vi "kf_update_p_k.vi"(11 "KF in":T2 {"K" format="%#_3g"; "y lim" format="%#_3g"; "x lim" format="%#_3g"; "P" format="%#_3g"; "H" format="%#_3g"; "x" format="%#_3g"; "Q" format="%#_3g"; "R" format="%#_3g"; "B" format="%#_3g"; "A" format="%#_3g"}) -> (2 "K":T1, 3 "P":T1)   [LabVIEW 2014]
uses:
  kalman_filter.ctl
  <vilib>/Analysis/Matrix/Datatypes/RealMatrix.ctl
  <vilib>/Analysis/baseanly.llb/Real A x B.vi
  <vilib>/Analysis/Matrix/Numeric/Add/Add - RM,RM.vi
  <vilib>/Analysis/baseanly.llb/Real Inverse Matrix.vi
  <vilib>/Analysis/7linalg.llb/Create Special Real Matrix.vi
  <vilib>/Analysis/Matrix/Numeric/Subtract/Subtract - RM,RM.vi
  <vilib>/Analysis/NI_AALBase.lvlib
  <vilib>/Analysis/Matrix/NI_Matrix.lvlib
  <vilib>/Analysis/NI_AALPro.lvlib
panel:
  # "Compute updated state covariance estimate and Kalman gain.  This is only necessary while the filter is reaching steady state."
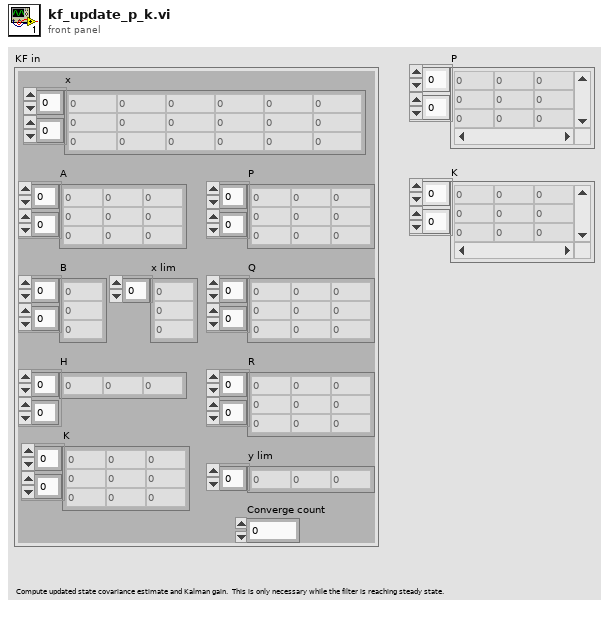
[diagram p1: front panel]
types:
  T1 = typedef "NI_Matrix.lvlib/RealMatrix.ctl" = dbl[][]
  T2 = typedef "kalman_filter.ctl" = cluster{"A":T1, "B":T1, "H":T1, "Q":T1, "R":T1, "x":T1, "P":T1, "x lim":dbl[], "y lim":dbl[], "K":T1, "Converge count":i32}
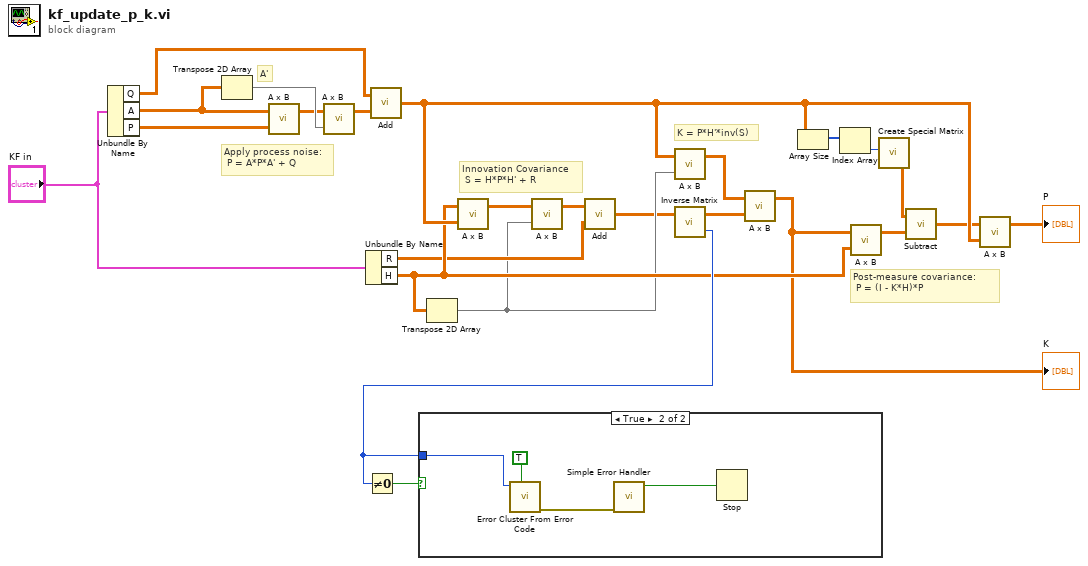
[diagram p0: block diagram]
diagram:
  # "Post-measure covariance:\n P = (I - K*H)*P"
  # "A'"
  # "K = P*H'*inv(S)"
  # "Innovation Covariance\n S = H*P*H' + R"
  # "Apply process noise:\n P = A*P*A' + Q"
  n1 = Unbundle By Name("KF in") -> ("Q"=w12:T1, "A"=w11:T1, "P"=w22:T1)
  n2 = Transpose 2D Array(2D array=w11) -> (transposed array=w3:T1)
  n3 = call-poly <vilib>:"A x B.vi"("B"=w22, "A"=w11) -> ("A x B"=w2:T1)  [unwired: 1 out]
  n4 = call-poly <vilib>:"A x B.vi"("B"=w3, "A"=w2) -> ("A x B"=w1:T1)  [unwired: 1 out]
  n5 = Unbundle By Name("KF in") -> ("R"=w19:T1, "H"=w20:T1)
  n6 = call-poly <vilib>:"Add.vi"("Real Matrix B"=w1, "Real Matrix A"=w12) -> ("A + B"=w21:T1)
  n7 = Transpose 2D Array(2D array=w20) -> (transposed array=w18:T1)
  n8 = call-poly <vilib>:"A x B.vi"("B"=w21, "A"=w20) -> ("A x B"=w4:T1)  [unwired: 1 out]
  n9 = call-poly <vilib>:"A x B.vi"("B"=w18, "A"=w4) -> ("A x B"=w5:T1)  [unwired: 1 out]
  n10 = call-poly <vilib>:"Add.vi"("Real Matrix B"=w19, "Real Matrix A"=w5) -> ("A + B"=w7:T1)
  n11 = call-poly <vilib>:"A x B.vi"("B"=w18, "A"=w21) -> ("A x B"=w6:T1)  [unwired: 1 out]
  n12 = call-poly <vilib>:"Inverse Matrix.vi"("Input Matrix"=w7) -> ("error"=w25:i32, "Inverse Matrix"=w8:T1)  [unwired: 1 in]
  n13 = Not Equal To 0?(x=w25) -> (x != 0?=w24:bool)
  n14 = case shown="True" w24 {
    tunnel: w25 -> [_ w29]
    frame False {
    }
    frame True {
      n15 = call <vilib>:"Error Cluster From Error Code.vi"("show call chain? (False)"=TRUE, "error code (0)"=w29) -> ("error out"=w27:errorcluster)  [unwired: 7 in]
      n16 = call <vilib>:"Simple Error Handler.vi"("error in (no error)"=w27) -> ("error?"=w26:bool)  [unwired: 4 in, 4 out]
      n17 = Stop(stop? (T)=w26) -> ()
    }
  }
  n18 = call-poly <vilib>:"A x B.vi"("B"=w8, "A"=w6) -> ("A x B"=w9:T1)  [unwired: 1 out]
  "K" <- w9
  n19 = Array Size(array=w21) -> (size(s)=w14:i32[])
  n20 = Index Array(array=w14) -> (element=w15:i32)  [unwired: 1 in]
  n21 = call-poly <vilib>:"A x B.vi"("B"=w20, "A"=w9) -> ("A x B"=w13:T1)  [unwired: 1 out]
  n22 = call-poly <vilib>:"Create Special Matrix.vi"("matrix size"=w15) -> ("Special Matrix"=w16:T1)  [unwired: 4 in, 1 out]
  n23 = call-poly <vilib>:"Subtract.vi"("Real Matrix B"=w13, "Real Matrix A"=w16) -> ("A - B"=w10:T1)
  n24 = call-poly <vilib>:"A x B.vi"("B"=w21, "A"=w10) -> ("A x B"=→"P":T1)  [unwired: 1 out]
